vi "enable_compression.vi"(7 "connection_reference":T1, 8 "error in (no error)":errorcluster, 10 "segment_column":string, 11 "hyper_table_name":string) -> (0 "error out":errorcluster)   [LabVIEW 2015, in "lv-timescaledb.lvlib"]
uses:
  lv-timescaledb.lvlib
  <vilib>/addons/database/Connection.llb/Conn ObjectReference.ctl
  <vilib>/addons/database/Command.llb/Cmd Execute.vi
  <vilib>/addons/database/Recordset.llb/Rec Destroy - Command.vi
  <vilib>/addons/database/Command.llb/Cmd Delete.vi
  <vilib>/addons/database/NI_Database_API.lvlib
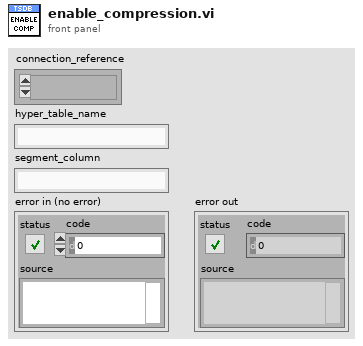
[diagram p1: front panel]
types:
  T1 = typedef "NI_Database_API.lvlib/Conn ObjectReference.ctl" = refnum<k1>
  T2 = typedef "NI_Database_API.lvlib/Cmd ObjectReference.ctl" = refnum<k1>
  T3 = typedef "NI_Database_API.lvlib/Cmd-Rec Object Reference.ctl" = refnum<k1>
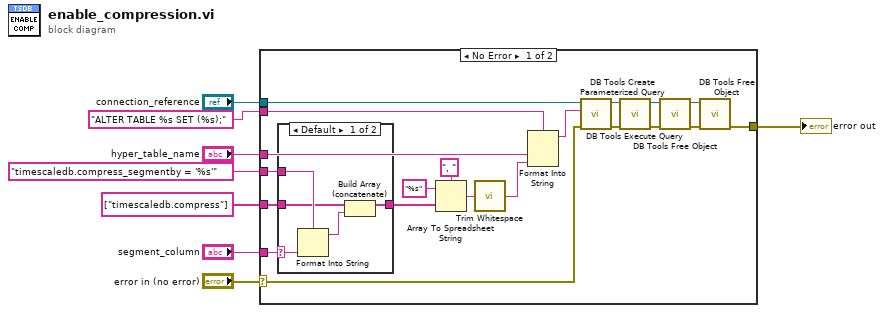
[diagram p0: block diagram]
diagram:
  n1 = case shown="No Error" "error in (no error)" {
    selector: "error in (no error)" -> [w18 w35]
    tunnel: "hyper_table_name" -> [w17 _]
    tunnel: "connection_reference" -> [w28 _]
    tunnel: [w27 w35] -> w6
    tunnel: "ALTER TABLE %s SET (%s);" -> [w20 _]
    tunnel: "segment_column" -> [w15 _]
    tunnel: "timescaledb.compress_segmentby = '%s'" -> [w14 _]
    tunnel: string[] ["timescaledb.compress"] -> [w9 _]
    frame No Error {
      n2 = case shown="Default" w15 {
        selector: w15 -> [w33 _]
        tunnel: w9 -> [w31 w34]
        tunnel: [w30 w34] -> w13
        tunnel: w14 -> [w32 _]
        frame Default {
          n3 = Format Into String(format string=w32, w33) -> (resulting string=w29:string)  [unwired: 2 in, 1 out]
          n4 = Build Array (concatenate)(w31, w29) -> (w30:string[])
        }
        frame "" {
        }
      }
      n5 = Array To Spreadsheet String(delimiter (Tab)=", ", array=w13, 3:"%s" ("format string")) -> (spreadsheet string=w16:string)
      n6 = call <vilib>:"Trim Whitespace.vi"("string"=w16) -> ("trimmed string"=w10:string)  [unwired: 1 in]
      n7 = Format Into String(format string=w20, w17, w10) -> (resulting string=w19:string)  [unwired: 2 in, 1 out]
      n8 = call <vilib>:"DB Tools Create Parameterized Query.vi"("error in (no error)"=w18, "SQL query"=w19, "connection reference"=w28) -> ("error out"=w25:errorcluster, "command reference"=w23:T2)  [unwired: 4 in, 1 out]
      n9 = call-poly <vilib>:"DB Tools Execute Query.vi"("error in (no error)"=w25, "command reference"=w23) -> ("error out"=w26:errorcluster, "command-recordset reference"=w22:T3)  [unwired: 6 in]
      n10 = call-poly <vilib>:"DB Tools Free Object.vi"("error in (no error)"=w26, "command-recordset reference"=w22) -> ("error out"=w24:errorcluster, "command reference"=w21:T2)  [unwired: 8 in]
      n11 = call-poly <vilib>:"DB Tools Free Object.vi"("error in (no error)"=w24, "command reference"=w21) -> ("error out"=w27:errorcluster)  [unwired: 8 in, 1 out]
    }
    frame Error {
    }
  }
  "error out" <- w6
